vi "niDTS BT LE Rx Test Configure.vi"(0 "Dummy Test Handle In":T6, 7 "BT LE Parameters":T1={"Channel"=0, "Tx Power (dBm)"=0.0, "External Attenuation (dB)"=0.0, "Payload Data"=enum."00001111", "Carrier Mode"=enum."Burst", "Number of Packets"=4, "Corrupt Alternate CRC"=FALSE, "Dirty Tx"=FALSE, "Payload Header"={"Length (-1 AutoSet Max)"=0}, "Trigger"={"TriggerEdge"=enum."RISing", "TriggerSource"=enum."IMMediate", "TriggerDelay (sec)"=0.0, "TriggerTimeout (sec)"=0.0}}, 9 "Result Index":i32, 11 "error in (no error)":errorcluster) -> (4 "Dummy Test Handle Out":T6, 15 "error out":errorcluster)   [LabVIEW 2014, in "niDTS BT.lvlib"]
uses:
  niDTS BT.lvlib
  BDR Tx Test/Includes/niDTS BT Rx Test INC Handle.ctl
  Rx Test/Objects/BASE_class/niDTS BT Rx Test.lvclass
  Includes/niDTS BT LE Rx Test INC Parameters.ctl
  Tx Test/Includes/niDTS BT Tx Test INC BD Payload Data.ctl
  Rx Test/Includes/niDTS BT Rx Test INC Carrier Mode.ctl
  Rx Test/Includes/niDTS BT Rx Test INC LE Payload Length.ctl
  Includes/niDTS BT DUT INC SG Trigger.ctl
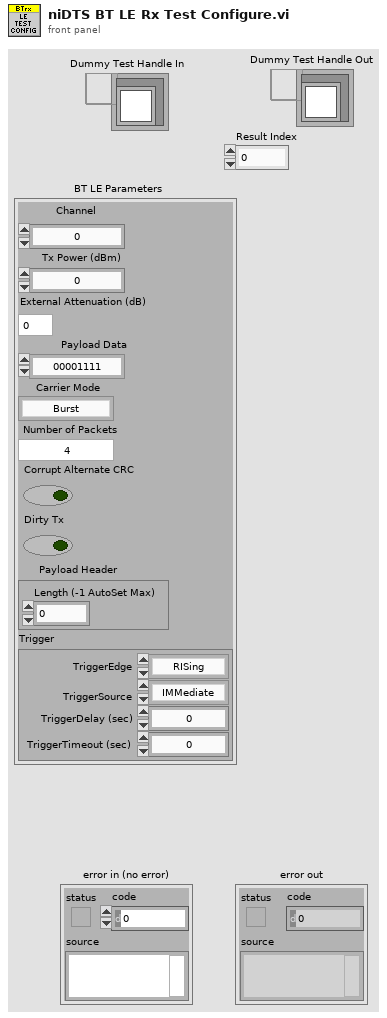
[diagram p1: front panel]
types:
  T1 = typedef "niDTS BT.lvlib/niDTS BT LE Rx Test INC Parameters.ctl" = cluster{"Channel":i32, "Tx Power (dBm)":dbl, "External Attenuation (dB)":dbl, "Payload Data":T2, "Carrier Mode":T3, "Number of Packets":i32, "Corrupt Alternate CRC":bool, "Dirty Tx":bool, "Payload Header":T4, "Trigger":T5}
  T2 = typedef "niDTS BT.lvlib/niDTS BT Tx Test INC BD Payload Data.ctl" = enum16{"0", "1", "01", "00001111", "PN9", "AUTO"}
  T3 = typedef "niDTS BT.lvlib/niDTS BT Rx Test INC Carrier Mode.ctl" = enum16{"Burst", "Continuous"}
  T4 = typedef "niDTS BT.lvlib/niDTS BT Rx Test INC LE Payload Length.ctl" = cluster{"Length (-1 AutoSet Max)":i32}
  T5 = typedef "niDTS BT.lvlib/niDTS BT DUT INC SG Trigger.ctl" = cluster{"TriggerEdge":enum16{"RISing", "FALLing"}, "TriggerSource":enum16{"IMMediate", "PFI 0", "PFI 1", "RTSI 0", "RTSI 1", "RTSI 2", "RTSI 3", "RTSI 4", "RTSI 5", "RTSI 6", "RTSI 7", "PXI STAR", "Software"}, "TriggerDelay (sec)":dbl, "TriggerTimeout (sec)":dbl}
  T6 = typedef "niDTS BT.lvlib/niDTS BT Rx Test INC Handle.ctl" = refnum<data-value>
  T7 = typedef "niDTS BT.lvlib/niDTS BT Rx Test INC Parameters.ctl" = cluster{"Channel":i32, "Dut Tx Power":dbl, "External Attenuation (dB)":dbl[], "Data Rate":enum16{"1", "2", "3"}, "Packet type":T8, "Payload Data":T2, "Carrier Mode":T3, "Number of Packets":i32, "Report Period (ms)":dbl, "BD ADDRESS":i64, "Dirty Tx":bool, "Corrupt Alternate CRC":bool, "Packet Header":T9, "Payload Header":T10, "Trigger":T5}
  T8 = typedef "niDTS BT.lvlib/niDTS BT INC Packet Type.ctl" = enum16{"NULL", "POLL", "FHS", "DM1", "DH1", "HV1", "HV2", "HV3", "EV3", "DV", "AUX1", "DM3", "DH3", "EV4", "EV5", "DM5", "DH5", "LE-TP"}
  T9 = typedef "niDTS BT.lvlib/niDTS BT Rx Test INC Packet Header.ctl" = cluster{"LT Address":i8, "Flow":i8, "ARQN":enum16{"NAK", "ACK"}, "Sequence Bit":i8}
  T10 = typedef "niDTS BT.lvlib/niDTS BT Rx Test INC Payload Header.ctl" = cluster{"LCh":i32, "HeaderFlowControlBit":bool, "Length (-1 AutoSet Max)":i32}
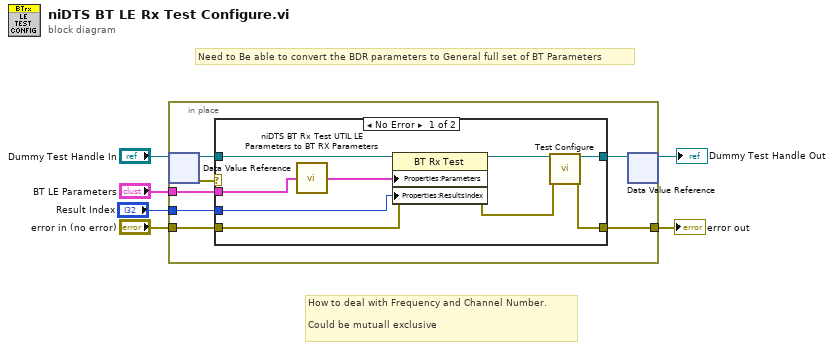
[diagram p0: block diagram]
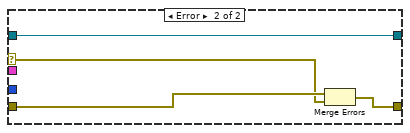
[diagram p2: hidden frame]
diagram:
  # "Need to Be able to convert the BDR parameters to General full set of BT Parameters"
  # "How to deal with Frequency and Channel Number.\n\nCould be mutuall exclusive"
  n1 = in-place {
    in-place-border: "error in (no error)" -> [w10]
    in-place-border: [w9] -> w5
    in-place-border: "BT LE Parameters" -> [w8]
    in-place-border: "Result Index" -> [w7]
    n2 = in-place-dvr #1("Dummy Test Handle In") -> (w12:refnum<class "niDTS BT Rx Test.lvclass">, w13:errorcluster)
    n3 = case shown="No Error" w13 {
      selector: w13 -> [_ w24]
      tunnel: w12 -> [w22 w26]
      tunnel: [w18 w26] -> w11
      tunnel: w10 -> [w21 w25]
      tunnel: [w19 w23] -> w9
      tunnel: w8 -> [w16 _]
      tunnel: w7 -> [w14 _]
      frame No Error {
        n4 = call "niDTS BT Rx Test UTIL LE Parameters to BT RX Parameters.vi"("BT LE Parameters"=w16) -> ("BT Rx Parameters"=w15:T7)  [unwired: 14 in]
        n5 = property class="BT Rx Test"(reference=w22, error in=w21, "Properties:Parameters"=w15, "Properties:ResultsIndex"=w14) -> (reference out=w17:refnum<class "niDTS BT Rx Test.lvclass">, error out=w20:errorcluster)
        n6 = call-dynamic "Test Configure.vi"("niDTS BT Rx Test in"=w17, "error in (no error)"=w20) -> ("niDTS BT Rx Test out"=w18:refnum<class "niDTS BT Rx Test.lvclass">, "error out"=w19:errorcluster)  [unwired: 12 in]
      }
      frame Error {
        n7 = Merge Errors(w25, w24) -> (w23:errorcluster)
      }
    }
    n8 = in-place-dvr #1(w11) -> (→"Dummy Test Handle Out":T6)  [unwired: 1 out]
  }
  "error out" <- w5
